vi "Classify Error.vi"(8 "Error to Classify":errorcluster, 11 "String":string) -> (0 "Classified Error":errorcluster)   [LabVIEW 2017]
doc: "This VI includes a \"classification\" that helps to identify an error. Classification is typically done by a Specific Error Handler, but can be done manually using this VI. Classifications are typically consumed by a Central Error Handler. Classifications are represented by appending information to the error's source string."
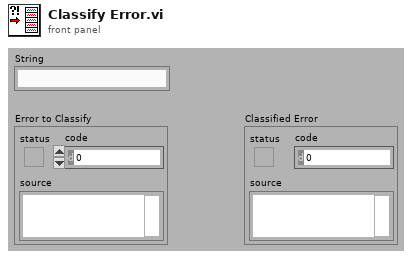
[diagram p1: front panel]
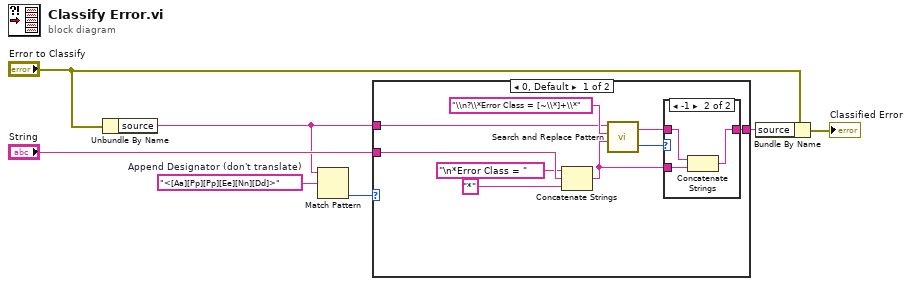
[diagram p0: block diagram]
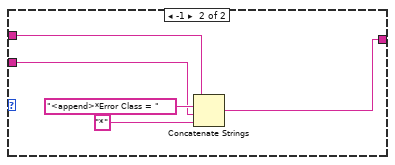
[diagram p3: hidden frame]
diagram:
  w4 = "<[Aa][Pp][Pp][Ee][Nn][Dd]>"  # Append Designator (don't translate)
  n1 = Unbundle By Name("Error to Classify") -> ("source"=w2:string)
  n2 = Match Pattern(string=w2, regular expression=w4) -> (offset past match=w3:i32)  [unwired: 4 out]
  n3 = case shown="0, Default" w3 {
    tunnel: [w16 w21] -> w7
    tunnel: "String" -> [w12 w23]
    tunnel: w2 -> [w8 w22]
    frame 0, Default {
      n4 = Concatenate Strings("\n*Error Class = " ("string"), w12, "*" ("string")) -> (w9:string)
      n5 = call <vilib>:"Search and Replace Pattern.vi"("string"=w8, "regular expression (\"\")"="\\n?\\*Error Class = [~\\*]+\\*" ("regular expression (\"\")"), "replace string (\"\")"=w9) -> ("result string"=w15:string, "offset past match"=w14:i32)  [unwired: 2 out]
      n6 = case shown="-1" w14 {
        tunnel: w15 -> [w17 w18]
        tunnel: [w17 w20] -> w16
        tunnel: w9 -> [_ w19]
        frame 0, Default {
        }
        frame -1 {
          n7 = Concatenate Strings(w18, w19) -> (w20:string)
        }
      }
    }
    frame -1 {
      n8 = Concatenate Strings(w22, "<append>*Error Class = " ("string"), w23, "*" ("string")) -> (w21:string)
    }
  }
  n9 = Bundle By Name(cluster="Error to Classify", "source"=w7) -> (→"Classified Error":errorcluster)
